vi "DensityCalculation.vi"(3 "dens":sgl[][](array[numeric]), 4 "bw image":T1) -> (0 "dens output":sgl[][](array[numeric]))   [LabVIEW 2015]
uses:
  <vilib>/vision/Image Controls.llb/IMAQ Image.ctl
  Realse/PlantType.dll
panel:
  in  "GridSize":i32=5
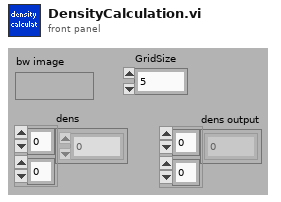
[diagram p1: front panel]
types:
  T1 = typedef "IMAQ Image.ctl" = refnum<image>
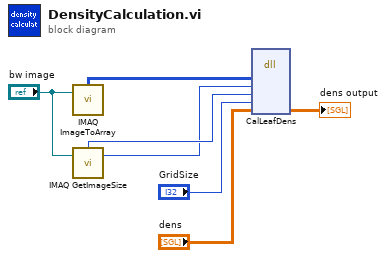
[diagram p0: block diagram]
diagram:
  n1 = call "IMAQ ImageToArray"("Image"="bw image") -> ("Image Pixels (U8)"=w6:u8[][])  [unwired: 2 in, 5 out]
  n2 = call "IMAQ GetImageSize"("Image"="bw image") -> ("Y Resolution"=w1:i32, "X Resolution"=w2:i32)  [unwired: 1 in, 3 out]
  n3 = dll-call lib="PTH2fabs E文章投稿&51. 代明球老师-玉米胁迫实验\tRGB程序maizeRealse\nPlantType.dll" fn="CalLeafDens"("bw"=w6, "row"=w1, "col"=w2, "GridSize"="GridSize", "dens"="dens") -> ("dens"=→"dens output":sgl[][])  [unwired: 7 in, 3 out]
